vi "Stacked Shift Registers.vi"() -> ()   [LabVIEW 2019]
panel:
  out "Previous Previous Number":dbl
  out "Sequentially Greater":bool
  out "Previous Number":dbl
  in  "stop":bool
  out "Random Number":dbl
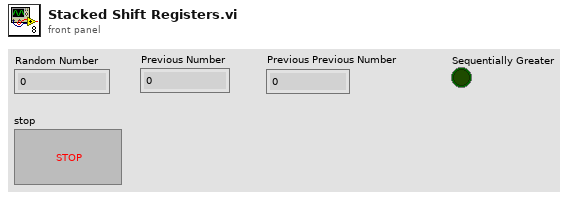
[diagram p1: front panel]
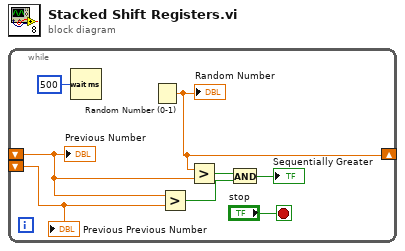
[diagram p0: block diagram]
diagram:
  n1 = while {
    shift-right: [w6] -> _
    shift-left: _ -> [w5]
    shift-left: _ -> [w4]
    stop <- "stop" stop-if-true
    n2 = Wait (ms)(milliseconds to wait=u32 500) -> ()  [unwired: 1 out]
    n3 = Random Number (0-1)() -> (number: 0 to 1=w6:dbl)
    "Random Number" <- w6
    n4 = Greater?(x=w5, y=w4) -> (0:w2:bool)
    n5 = Greater?(x=w6, y=w5) -> (0:w3:bool)
    n6 = And(x=w3, y=w2) -> (x .and. y?=→"Sequentially Greater":bool)
    "Previous Number" <- w5
    "Previous Previous Number" <- w4
  }
